vi "Source Limit.vi"(6 "Limit (0.000)":dbl, 7 "Function (Current)":enum32{"Current", "Voltage"}(ring), 8 "error in (no error)":errorcluster, 9 "Channel (Channel A)":T1, 10 "Node In":string, 11 "VISA resource name":refnum<visa-resource-name>) -> (0 "error out":errorcluster, 2 "Node Out":string, 3 "VISA resource name out":refnum<visa-resource-name>, 4 "Command String":string)   [LabVIEW 2013, in "Keithley 2600 Series.lvlib"]
doc: "This VI sets the SMU Source Limit.\n\nThe limit will stop the source from sourcing at the configured output level if it would require the SMU to source above the limit level.\n\nWhen sourcing current, use the limit to limit the voltage output of the source. When sourcing voltage, use the limit to limit the current output of the source.\n\n<b>Functions and Attributes Used</b>\nsmuX.source.limitY"
uses:
  Keithley 2600 Series.lvlib
  Private/GlobalVariables.vi
  Channel.ctl
panel:
  # "(c) 2008 Keithley Instruments, Inc.  ALL RIGHTS RESERVED."
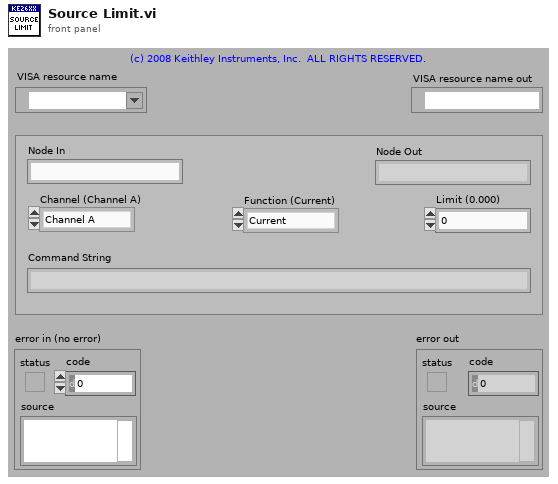
[diagram p1: front panel]
types:
  T1 = typedef "Keithley 2600 Series.lvlib/Channel.ctl" = enum32{"Channel A", "Channel B"}
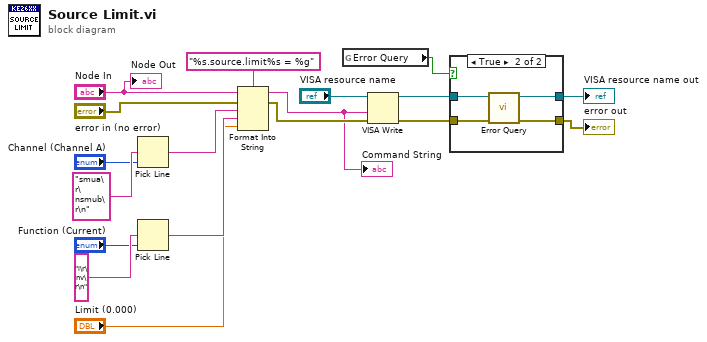
[diagram p0: block diagram]
diagram:
  n1 = Pick Line(multi-line string="smua\r\nsmub\r\n" ("options"), line index="Channel (Channel A)") -> (output string=w6:string)  [unwired: 1 out]
  n2 = Pick Line(multi-line string="i\r\nv\r\n" ("options"), line index="Function (Current)") -> (output string=w5:string)  [unwired: 1 out]
  n3 = Format Into String(format string="%s.source.limit%s = %g", initial string="Node In", error in="error in (no error)", w6, w5, "Limit (0.000)") -> (resulting string=w1:string, error out=w2:errorcluster)
  "Command String" <- w1
  n4 = global read "GlobalVariables.vi" "Error Query"() -> (w14:bool)
  n5 = VISA Write(VISA resource name="VISA resource name", write buffer=w1, error in (no error)=w2) -> (VISA resource name out=w13:refnum<visa-resource-name>, error out=w12:errorcluster)  [unwired: 1 out]
  n6 = case shown="True" w14 {
    tunnel: w13 -> [w20 w24]
    tunnel: w12 -> [w19 w23]
    tunnel: [w20 w22] -> w11
    tunnel: [w19 w21] -> w10
    frame False {
    }
    frame True {
      n7 = call "Error Query.vi"("error in (no error)"=w23, "VISA resource name"=w24) -> ("error out"=w21:errorcluster, "VISA resource name out"=w22:refnum<visa-resource-name>)  [unwired: 8 out]
    }
  }
  "VISA resource name out" <- w11
  "error out" <- w10
  "Node Out" <- "Node In"
